vi "Write Spark Trigger Number.vi"(8 "error in (no error)":errorcluster, 10 "Spark Trigger Index":i32, 11 "PulseData in":refnum<class "PulseData.lvclass">) -> (0 "error out":errorcluster, 3 "PulseData out":refnum<class "PulseData.lvclass">)   [LabVIEW 2013, in "Controls Log Monitor.lvlib" / "PulseData.lvclass"]
uses:
  PulseData.lvclass
  PulseData.lvclass/PulseData.ctl
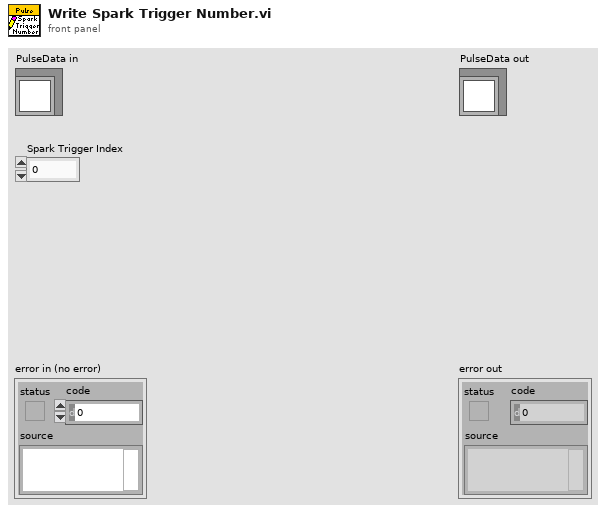
[diagram p1: front panel]
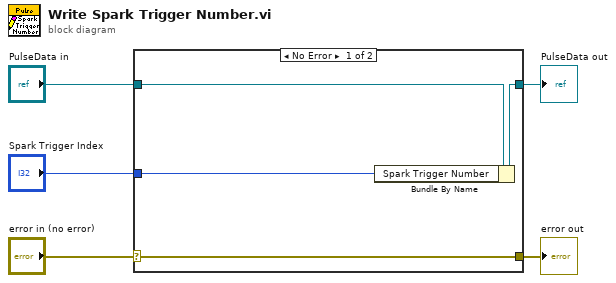
[diagram p0: block diagram]
diagram:
  n1 = case shown="No Error" "error in (no error)" {
    selector: "error in (no error)" -> [w9 w10]
    tunnel: [w9 w10] -> w4
    tunnel: [w7 w11] -> w2
    tunnel: "PulseData in" -> [w8 w11]
    tunnel: "Spark Trigger Index" -> [w6 _]
    frame No Error {
      n2 = Bundle By Name(cluster=w8, "Spark Trigger Number"=w6) -> (w7:refnum<class "PulseData.lvclass">)
    }
    frame Error {
    }
  }
  "error out" <- w4
  "PulseData out" <- w2
